vi "Check and Override Channel Configuration.vi"(8 "error in (no error)":errorcluster, 10 "Custom Config Data in":u8[](array[numeric]) format="%.0x", 11 "CIF_NIChn_FIFO_DAQ in":refnum<class "CIF_NIChn_DAQ_Base.lvclass">) -> (0 "error out":errorcluster, 2 "Custom Config Data out":u8[](array[numeric]) format="%.0x", 3 "CIF_NIChn_FIFO_DAQ out":refnum<class "CIF_NIChn_DAQ_Base.lvclass">)   [LabVIEW 2021, in "CIF_NIChn_DAQ_Base.lvclass"]
uses:
  CIF_NIChn_DAQ_Base.lvclass
  <vilib>/CIF Foundation/CIF Utilities/DataTypes/Unflatten U64.vi
  <vilib>/CIF Foundation/CIF Utilities/DataTypes/Flatten U64.vi
  ChannelCommon/ChannelCommon.lvlib
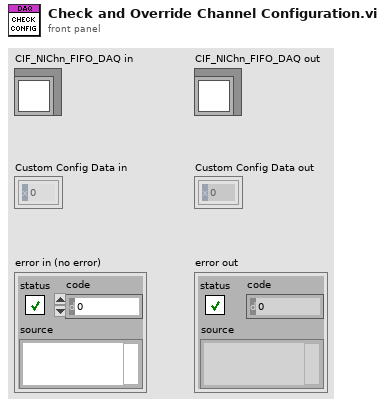
[diagram p1: front panel]
types:
  T1 = typedef "ChannelCommon.lvlib/FIFO Config.ctl" = cluster{"Max Bytes/Msg":u64, "Max Msg/FIFO":u64, "Flags":u64}
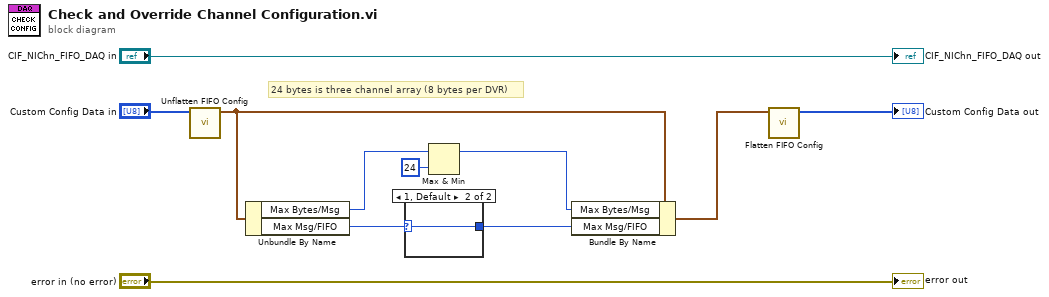
[diagram p0: block diagram]
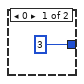
[diagram p2: hidden frame]
diagram:
  # "24 bytes is three channel array (8 bytes per DVR)"
  n1 = call "Unflatten FIFO Config.vi"("Flattened Data in"="Custom Config Data in") -> ("FIFO Config out"=w6:T1)  [unwired: 9 in, 1 out]
  n2 = Unbundle By Name(w6) -> ("Max Bytes/Msg"=w3:u64, "Max Msg/FIFO"=w5:u64)
  n3 = case shown="1, Default" w5 {
    selector: w5 -> [_ w13]
    tunnel: [u64 3 ("y") w13] -> w4
    frame 0 {
    }
    frame 1, Default {
    }
  }
  n4 = Max & Min(x=w3, y=u64 24) -> (max(x,y)=w1:u64)  [unwired: 1 out]
  n5 = Bundle By Name(cluster=w6, "Max Bytes/Msg"=w1, "Max Msg/FIFO"=w4) -> (w7:T1)
  n6 = call "Flatten FIFO Config.vi"("FIFO Config in"=w7) -> ("Flattened FIFO Config"=→"Custom Config Data out":u8[])  [unwired: 10 in]
  "error out" <- "error in (no error)"
  "CIF_NIChn_FIFO_DAQ out" <- "CIF_NIChn_FIFO_DAQ in"
